vi "GenerateStageCoordinatesForMap.vi"(8 "error in (no error)":errorcluster) -> (0 "error out":errorcluster, 3 "Stage Coordinates for Map":cluster{"X":sgl, "Y":sgl}[](array[cluster]))   [LabVIEW 2017]
doc: "Use this template to build a VI to use as a subVI."
uses:
  Microscope/MicroscopeControllerEnum.ctl
  AEROTECstageAPI/StageEnum.ctl
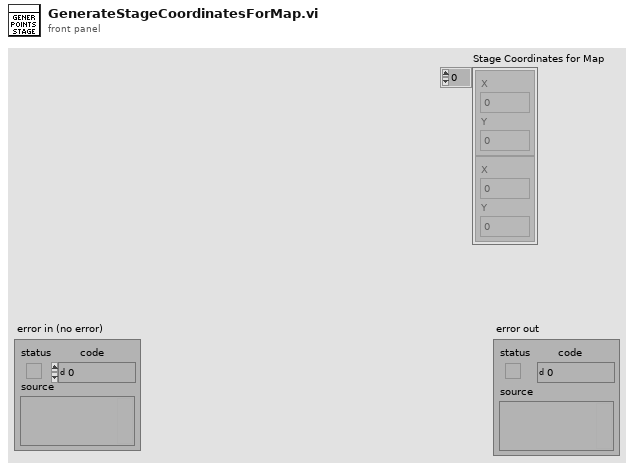
[diagram p1: front panel]
types:
  T1 = typedef "StageEnum.ctl" = enum16{"Get Current Pos!", "Move axis!", "Enable Stage!", "Stop Stage Controller!", "Set Default Speeds!", "Get Stage Parameters", "Start Stage Controller!", "Init", "Go Home!"}
  T2 = typedef "MicroscopeControllerEnum.ctl" = enum16{"Init!", "Start!", "Stop!", "GetMicroscopeVIRef", "CalculateRelPointForStagemicrons", "InsertCallbackEvent!", "InsertLaserPoint!", "InsertMapPoints!", "InsertMicroscopeImageRef!"}
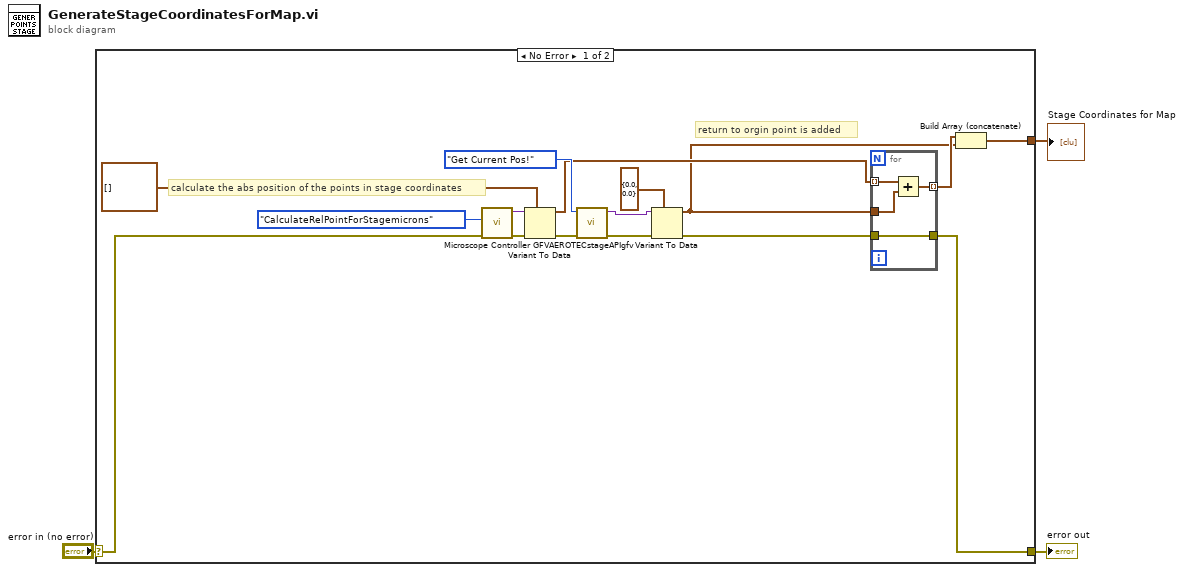
[diagram p0: block diagram]
diagram:
  n1 = case shown="No Error" "error in (no error)" {
    selector: "error in (no error)" -> [w6 w24]
    tunnel: [w5 w24] -> w2
    tunnel: [w4 _] -> w1
    frame No Error {
      # "return to orgin point is added"
      # "calculate the abs position of the points in stage coordinates"
      n2 = call "Microscope Controller GFV.vi"("error in (no error)"=w6, "MicroscopeEnum"=MicroscopeControllerEnum."CalculateRelPointForStagemicrons") -> ("error out"=w19:errorcluster, "Data Out"=w17:variant)  [unwired: 8 in]
      n3 = Variant To Data(error in=w19, type=cluster{"X":sgl, "Y":sgl}[] [] ("Array of Real World Coordinates"), Variant=w17) -> (data=w10:cluster{"X":sgl, "Y":sgl}[], error out=w15:errorcluster)
      n4 = call "AEROTECstageAPIgfv.vi"("error in (no error)"=w15, "StageContrlEnum"=StageEnum."Get Current Pos!") -> ("error out"=w12:errorcluster, "Data Out"=w13:variant)  [unwired: 8 in]
      n5 = Variant To Data(error in=w12, type=cluster{"X":sgl, "Y":sgl} {"X"=0.0, "Y"=0.0}, Variant=w13) -> (data=w7:cluster{"X":sgl, "Y":sgl}, error out=w9:errorcluster)
      n6 = for {
        tunnel: w10 -> [w22] mode=indexing
        tunnel: w7 -> [w21]
        tunnel: [w23] -> w5
        tunnel: w9 -> [w23]
        tunnel: [w20] -> w8 mode=indexing
        n7 = Add(x=w22, y=w21) -> (x+y=w20:cluster{"X":sgl, "Y":sgl})
      }
      n8 = Build Array (concatenate)(w8, w7) -> (w4:cluster{"X":sgl, "Y":sgl}[])
    }
    frame Error {
    }
  }
  "error out" <- w2
  "Stage Coordinates for Map" <- w1
